vi "Device.Init.vi"(8 "error in (no error)":errorcluster, 11 "OPA.OrpheusHP in":refnum<class "OPA.OrpheusHP.lvclass">) -> (0 "error out":errorcluster, 2 "Result":bool, 3 "OPA.OrpheusHP out":refnum<class "OPA.OrpheusHP.lvclass">)   [LabVIEW 2017, in "OPA.OrpheusHP.lvclass"]
uses:
  OPA.OrpheusHP.lvclass
  D:/upwork/Laser Measurement Tool/Laser/project/Subsystems/OPA/OPA.lvclass
  Typedefs/Resource--Cluster.ctl
  D:/upwork/Laser Measurement Tool/Topas4PublicAPI/NET_SDK/Topas4Lib.dll
  Topas4PublicAPI/NET_SDK/Topas4Lib.dll
  OPA/OPA.lvclass
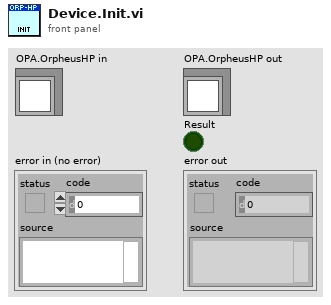
[diagram p1: front panel]
types:
  T1 = typedef "OPA.OrpheusHP.lvclass/Resource--Cluster.ctl" = cluster{"TopasDevice":refnum<k24>}
  T2 = typedef "OPA.lvclass/Configuration--Cluster.ctl" = cluster{"Serial Number":string}
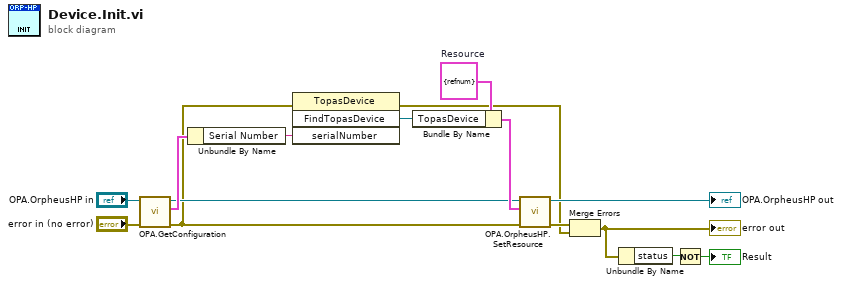
[diagram p0: block diagram]
diagram:
  w11 = T1 {"TopasDevice"=refnum}  # Resource
  n1 = call "OPA.GetConfiguration.vi"("error in (no error)"="error in (no error)", "OPA"="OPA.OrpheusHP in") -> ("error out"=w6:errorcluster, "Configuration"=w13:T2, "OPA out"=w8:refnum<class "OPA.OrpheusHP.lvclass">)  [unwired: 7 in]
  n2 = Unbundle By Name(w13) -> ("Serial Number"=w12:string)
  n3 = invoke class="TopasDevice" method="FindTopasDevice"(error in=w6, "serialNumber"=w12) -> (error out=w4:errorcluster, "FindTopasDevice"=w10:refnum<k24>)  [unwired: 2 in, 2 out]
  n4 = Bundle By Name(cluster=w11, "TopasDevice"=w10) -> (w9:T1)
  n5 = call "OPA.OrpheusHP.SetResource.vi"("error in (no error)"=w6, "Resource"=w9, "OPA.OrpheusHP in"=w8) -> ("error out"=w5:errorcluster, "OPA.OrpheusHP out"=→"OPA.OrpheusHP out":refnum<class "OPA.OrpheusHP.lvclass">)  [unwired: 7 in]
  n6 = Merge Errors(w5, w4) -> (w3:errorcluster)
  "error out" <- w3
  n7 = Unbundle By Name(w3) -> ("status"=w2:bool)
  n8 = Not(x=w2) -> (.not. x?=→"Result":bool)
